vi "Dashboard Loop.vi"(11 "connection ID":refnum<k16>) -> ()   [LabVIEW 2017]
uses:
  Common Code/Dashboard Status Data.ctl
  Common Code/Elevator Status Cluster.ctl
  Common Code/Elevator State.ctl
  Common Code/Elevator Mode.ctl
  Common Code/Drivetrain Status Cluster.ctl
  Common Code/Drivetrain Mode.ctl
  Common Code/DT Encoder Values.ctl
  Common Code/Intake Status Cluster.ctl
  Common Code/Intake Mode.ctl
  Common Code/Intake States.ctl
  Common Code/Climb Status Cluster.ctl
  Common Code/Intake PDP Info.ctl
  Common Code/Auton Command Cluster.ctl
  Common Code/Robot Info.ctl
  <vilib>/Rock Robotics/WPI/DriverStation/WPI_DriverStationAllianceInfo.ctl
  <vilib>/Rock Robotics/WPI/DriverStation/WPI_DriverStationPositionInfo.ctl
  <vilib>/Rock Robotics/WPI/DriverStation/WPI_DriverStationRobotMode2.ctl
  Common Code/Camera.ctl
  <vilib>/vision/Image Controls.llb/IMAQ Image.ctl
  Robot Global Data.vi
panel:
  out "Length":dbl
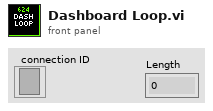
[diagram p1: front panel]
types:
  T1 = typedef "Dashboard Status Data.ctl" = cluster{"Elevator Status Cluster":T2, "Drivetrain Status Cluster":T5, "Intake Status Cluster":T8, "Climb Status Cluster":T11, "Intake PDP Info":T12, "Auton Command Cluster":T13, "Pressure ":dbl, "Auton Field Index":i32, "Auton File Index":i32, "Auton Side Index":i32, "Auton Side":string, "Field Config":string, "Robot Info":T14, "Camera":T18}
  T2 = typedef "Elevator Status Cluster.ctl" = cluster{"Finished":bool, "Elevator Power":dbl, "Elevator State":T3, "Elevator Mode":T4, "Elevator Height":dbl, "At Bottom?":bool, "At Top?":bool, "Scale high?":bool, "PID Output":dbl, "2nd Gear":bool}
  T3 = typedef "Elevator State.ctl" = enum16{"Idle", "Ground", "Mid", "Scale", "Switch"}
  T4 = typedef "Elevator Mode.ctl" = enum16{"Semi Auto", "Manual", "Auto"}
  T5 = typedef "Drivetrain Status Cluster.ctl" = cluster{"Throttle (Y)":dbl, "Steer (X)":dbl, "Drivetrain Mode":T6, "Brake?":bool, "Distance Drive Complete?":bool, "PID Drive Complete?":bool, "Creep Mode?":bool, "Gyro Steer Complete?":bool, "Gyro":dbl, "Heading Target":dbl, "Distance Target":dbl, "2nd Gear":bool, "Drivetrain Encoder Values":T7}
  T6 = typedef "Drivetrain Mode.ctl" = enum16{"Manual", "Gyro Steer", "PID Drive", "Distance Drive", "Autonomous"}
  T7 = typedef "DT Encoder Values.ctl" = cluster{"Left Encoder":cluster{"Distance":dbl, "Speed":dbl, "Tick":dbl}, "Right Encoder":cluster{"Distance":dbl, "Speed":dbl, "Tick":dbl}}
  T8 = typedef "Intake Status Cluster.ctl" = cluster{"Intake Mode":T9, "Intake States":T10, "Intake Current Angle":dbl, "Cube In Posession?":bool, "Intake Wrist Up?":bool, "Right Roller Power":dbl, "Angle Power":dbl, "Left Roller Power":dbl}
  T9 = typedef "Intake Mode.ctl" = enum16{"Auto", "Semi Auto", "Manual"}
  T10 = typedef "Intake States.ctl" = enum16{"Zero", "Override Angle", "Idle", "Drop Mid", "Drop Low", "Outtake", "Intake"}
  T11 = typedef "Climb Status Cluster.ctl" = cluster{"Climb":bool, "Time Remaining":dbl, "Button Pressed":bool}
  T12 = typedef "Intake PDP Info.ctl" = cluster{"Voltage Percent Output":dbl, "Output Voltage":dbl, "Bus Voltage":dbl, "Device ID":dbl, "Output Current":dbl, "Sensor Velocity":dbl, "Sensor Position":dbl, "Pulse Width Position":dbl, "Pulse Width Velocity":dbl, "Temperature":dbl, "Inverted?":bool}
  T13 = typedef "Auton Command Cluster.ctl" = cluster{"commandID":dbl, "headingTarget":dbl, "async":dbl, "elevatorCommand":dbl, "intakeMode":dbl, "maxTime":dbl, "ySpeed":dbl, "zeroGyro":dbl, "intakeCommand":dbl, "distanceTarget":dbl, "xSpeed":dbl, "elevatorMode":dbl, "scaleHigh":dbl, "rollerSpeed":dbl, "intakeAngle":dbl, "manualOpen":dbl, "secondGear":dbl, "elevatorPower":dbl, "waitFor":dbl}
  T14 = typedef "Robot Info.ctl" = cluster{"FMS":bool, "Switch and Scale Sides":string, "Event Name":string, "Alliance":T15, "Position":T16, "Match Number":u16, "Robot Mode":T17, "Match Time(s)":sgl}
  T15 = typedef "WPI_DriverStationAllianceInfo.ctl" = enum16{"Red", "Blue", "Invalid"}
  T16 = typedef "WPI_DriverStationPositionInfo.ctl" = enum16{"1", "2", "3"}
  T17 = typedef "WPI_DriverStationRobotMode2.ctl" = enum16{"Autonomous Disabled", "Autonomous Enabled", "Teleop Disabled", "Teleop Enabled", "Disconnected", "Finish", "Test Disabled", "Test Enabled", "Emergency Stopped"}
  T18 = typedef "Camera.ctl" = cluster{"Front Camera Display":T19}
  T19 = typedef "IMAQ Image.ctl" = refnum<image>
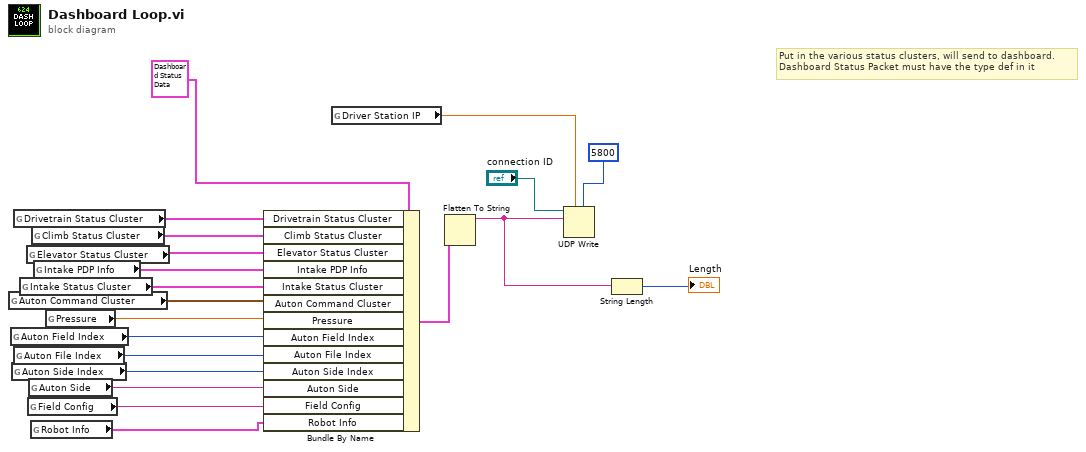
[diagram p0: block diagram]
diagram:
  # "Put in the various status clusters, will send to dashboard.\nDashboard Status Packet must have the type def in it"
  n1 = global read "Robot Global Data.vi" "Auton Command Cluster"() -> (w9:T13)
  n2 = global read "Robot Global Data.vi" "Auton Field Index"() -> (w7:i32)
  n3 = global read "Robot Global Data.vi" "Auton Side Index"() -> (w5:i32)
  n4 = global read "Robot Global Data.vi" "Drivetrain Status Cluster"() -> (w15:T5)
  n5 = global read "Robot Global Data.vi" "Auton File Index"() -> (w6:i32)
  n6 = global read "Robot Global Data.vi" "Intake Status Cluster"() -> (w11:T8)
  n7 = global read "Robot Global Data.vi" "Elevator Status Cluster"() -> (w13:T2)
  n8 = global read "Robot Global Data.vi" "Field Config"() -> (w3:string)
  n9 = global read "Robot Global Data.vi" "Auton Side"() -> (w4:string)
  n10 = global read "Robot Global Data.vi" "Robot Info"() -> (w2:T14)
  n11 = global read "Robot Global Data.vi" "Climb Status Cluster"() -> (w14:T11)
  n12 = global read "Robot Global Data.vi" "Intake PDP Info"() -> (w12:T12)
  n13 = global read "Robot Global Data.vi" "Pressure"() -> (w8:dbl)
  n14 = Bundle By Name(cluster=T1 {"Elevator Status Cluster"={"Finished"=FALSE, "Elevator Power"=0.0, "Elevator State"=enum."Idle", "Elevator Mode"=enum."Manual", "Elevator Height"=0.0, "At Bottom?"=FALSE, "At Top?"=FALSE, "Scale high?"=FALSE, "PID Output"=0.0, "2nd Gear"=FALSE}, "Drivetrain Status Cluster"={"Throttle (Y)"=0.0, "Steer (X)"=0.0, "Drivetrain Mode"=enum."Manual", "Brake?"=FALSE, "Distance Drive Complete?"=FALSE, "PID Drive Complete?"=FALSE, "Creep Mode?"=FALSE, "Gyro Steer Complete?"=FALSE, "Gyro"=0.0, "Heading Target"=0.0, "Distance Target"=0.0, "2nd Gear"=FALSE, "Drivetrain Encoder Values"={"Left Encoder"={"Distance"=0.0, "Speed"=0.0, "Tick"=0.0}, "Right Encoder"={"Distance"=0.0, "Speed"=0.0, "Tick"=0.0}}}, "Intake Status Cluster"={"Intake Mode"=enum."Manual", "Intake States"=enum."Zero", "Intake Current Angle"=0.0, "Cube In Posession?"=FALSE, "Intake Wrist Up?"=FALSE, "Right Roller Power"=0.0, "Angle Power"=0.0, "Left Roller Power"=0.0}, "Climb Status Cluster"={"Climb"=FALSE, "Time Remaining"=0.0, "Button Pressed"=FALSE}, "Intake PDP Info"={"Voltage Percent Output"=0.0, "Output Voltage"=0.0, "Bus Voltage"=0.0, "Device ID"=0.0, "Output Current"=0.0, "Sensor Velocity"=0.0, "Sensor Position"=0.0, "Pulse Width Position"=0.0, "Pulse Width Velocity"=0.0, "Temperature"=0.0, "Inverted?"=FALSE}, "Auton Command Cluster"={"commandID"=0.0, "headingTarget"=0.0, "async"=0.0, "elevatorCommand"=0.0, "intakeMode"=0.0, "maxTime"=0.0, "ySpeed"=0.0, "zeroGyro"=0.0, "intakeCommand"=0.0, "distanceTarget"=0.0, "xSpeed"=0.0, "elevatorMode"=0.0, "scaleHigh"=0.0, "rollerSpeed"=0.0, "intakeAngle"=0.0, "manualOpen"=0.0, "secondGear"=0.0, "elevatorPower"=0.0, "waitFor"=0.0}, "Pressure "=0.0, "Auton Field Index"=0, "Auton File Index"=0, "Auton Side Index"=0, "Auton Side"="", "Field Config"="", "Robot Info"={"FMS"=FALSE, "Switch and Scale Sides"="", "Event Name"="", "Alliance"=enum."Red", "Position"=enum."1", "Match Number"=0, "Robot Mode"=enum."Autonomous Disabled", "Match Time(s)"=0.0}, "Camera"={"Front Camera Display"=refnum}} ("Dashboard Status Data"), "Drivetrain Status Cluster"=w15, "Climb Status Cluster"=w14, "Elevator Status Cluster"=w13, "Intake PDP Info"=w12, "Intake Status Cluster"=w11, "Auton Command Cluster"=w9, "Pressure"=w8, "Auton Field Index"=w7, "Auton File Index"=w6, "Auton Side Index"=w5, "Auton Side"=w4, "Field Config"=w3, "Robot Info"=w2) -> (w20:T1)
  n15 = global read "Robot Global Data.vi" "Driver Station IP"() -> (w16:dbl)
  n16 = Flatten To String(anything=w20) -> (data string=w17:string)  [unwired: 3 in, 2 out]
  n17 = UDP Write(address=w16, port or service name=u16 5800, connection ID="connection ID", data in=w17) -> ()  [unwired: 2 in, 2 out]
  n18 = String Length(string=w17) -> (length=→"Length":i32)
